vi "TestBed_NET.vi"() -> ()   [LabVIEW 2018]
uses:
  System.Net.Http
  <vilib>/httpClient/LabVIEWHTTPClient.lvlib
  <vilib>/httpClient/MultipartData.ctl
  <vilib>/addons/_JKI.lib/REST Client/classes/REST Client/REST Client.lvclass
panel:
  out "Numeric":i32
  out "Array 2":cluster{"Array":string[]}[](array[cluster])
  in  "ProxyAddress":string
  in  "String":string="https://reqres.in/api/users?page=2"
  out "Array":string[](array[string])
  out "Result":string
  out "StatusCode":i32(ring)=100 items=["Continue"=100, "SwitchingProtocols"=101, "OK"=200, "Created"=201, "Accepted"=202, "NonAuthoritativeInformation"=203, "NoContent"=204, "ResetContent"=205, "PartialContent"=206, "MultipleChoices, Ambiguous"=300, "MovedPermanently, Moved"=301, "Found, Redirect"=302, "SeeOther, RedirectMethod"=303, "NotModified"=304, "UseProxy"=305, "Unused"=306, "TemporaryRedirect, RedirectKeepVerb"=307, "BadRequest"=400, "Unauthorized"=401, "PaymentRequired"=402, "Forbidden"=403, "NotFound"=404, "MethodNotAllowed"=405, "NotAcceptable"=406, "ProxyAuthenticationRequired"=407, "RequestTimeout"=408, "Conflict"=409, "Gone"=410, "LengthRequired"=411, "PreconditionFailed"=412, "RequestEntityTooLarge"=413, "RequestUriTooLong"=414, "UnsupportedMediaType"=415, "RequestedRangeNotSatisfiable"=416, "ExpectationFailed"=417, "UpgradeRequired"=426, "InternalServerError"=500, "NotImplemented"=501, "BadGateway"=502, "ServiceUnavailable"=503, "GatewayTimeout"=504, "HttpVersionNotSupported"=505]
  # "http://httpbin.org/#/"
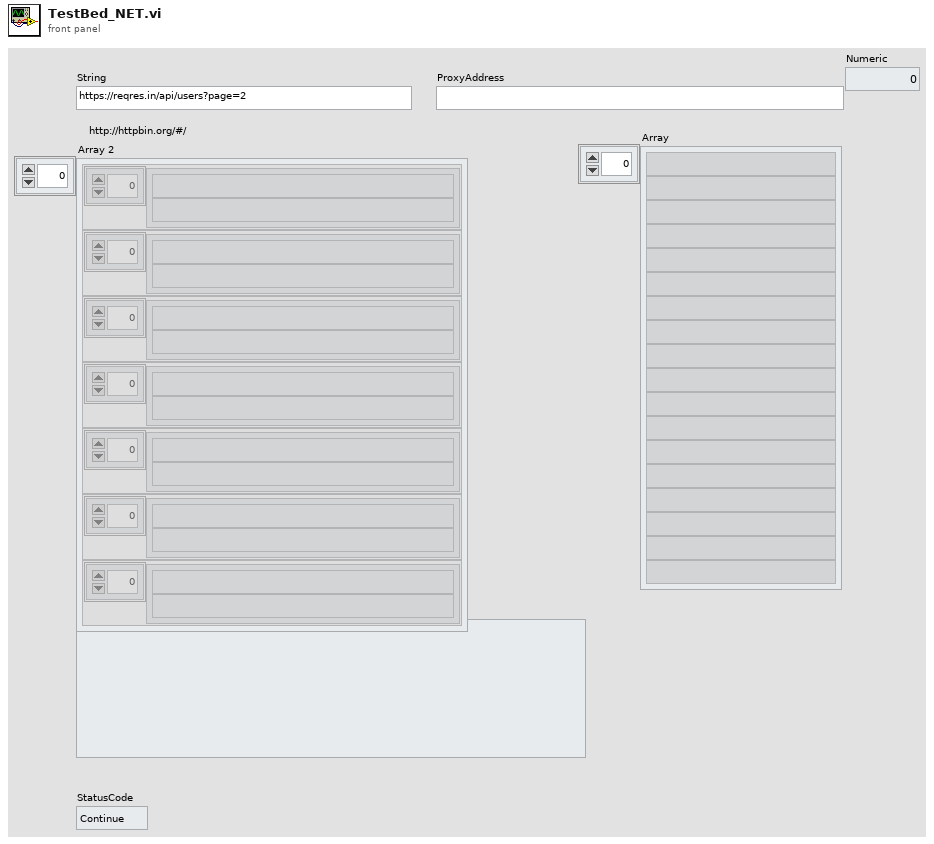
[diagram p1: front panel]
types:
  T1 = typedef "LabVIEWHTTPClient.lvlib/MultipartData.ctl" = cluster{"Name":string, "Value":string, "File":path, "Filename":string, "MIME type":string}
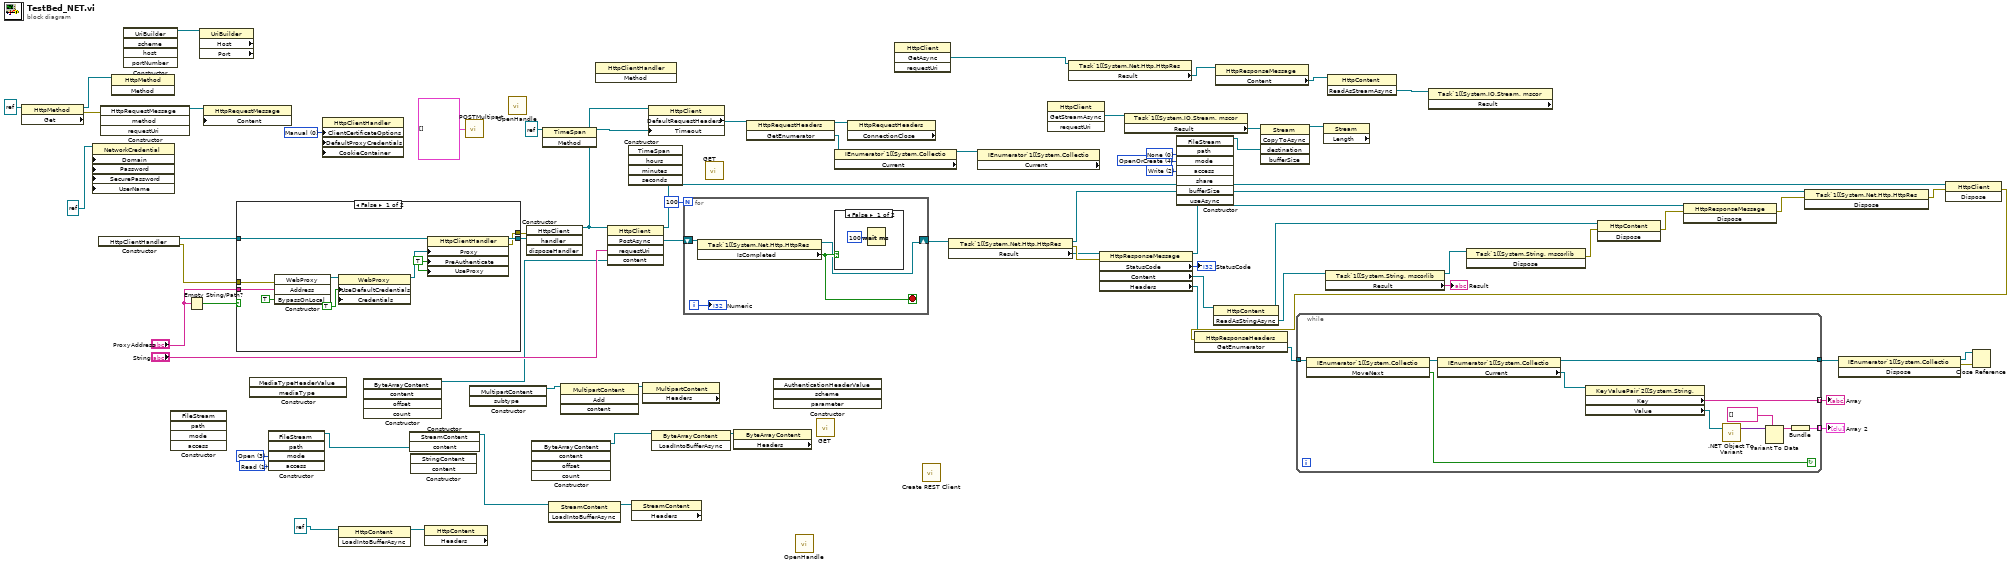
[diagram p0: block diagram]
diagram:
  w3 = 0 items=["None"=0, "Read"=1, "Write"=2, "ReadWrite"=3, "Delete"=4, "Inheritable"=16] ("share")
  w21 = 0 items=["Manual", "Automatic"] ("ClientCertificateOptions")
  w25 = 2 items=["Read"=1, "Write"=2, "ReadWrite"=3] ("access")
  w26 = 4 items=["CreateNew"=1, "Create"=2, "Open"=3, "OpenOrCreate"=4, "Truncate"=5, "Append"=6] ("mode")
  w31 = 1 items=["Read"=1, "Write"=2, "ReadWrite"=3] ("access")
  w32 = 3 items=["CreateNew"=1, "Create"=2, "Open"=3, "OpenOrCreate"=4, "Truncate"=5, "Append"=6] ("mode")
  n1 = property class="HttpMethod" props=["Get"](reference=refnum<k24> refnum) -> (reference out=w14:refnum<k24>, error out=w15:errorcluster)  [unwired: 1 in, 1 out]
  n2 = property class="NetworkCredential" props=["Domain", "Password", "SecurePassword", "UserName"](reference=refnum<k24> refnum ("cred")) -> ()  [unwired: 5 in, 2 out]
  n3 = constructor class="HttpClientHandler"() -> (reference out=w62:refnum<k24>, error out=w60:errorcluster)  [unwired: 3 in, 1 out]
  n4 = constructor class="HttpRequestMessage"(error in=w15) -> (reference out=w13:refnum<k24>)  [unwired: 4 in, 4 out]
  n5 = invoke class="HttpMethod" method=#-1(reference=w14) -> ()  [unwired: 2 in, 3 out]
  n6 = constructor class="UriBuilder"() -> (reference out=w6:refnum<k24>)  [unwired: 6 in, 5 out]
  n7 = constructor class="FileStream"() -> ()  [unwired: 6 in, 6 out]
  n8 = Empty String/Path?(string/path="ProxyAddress") -> (empty?=w58:bool)
  n9 = property class="UriBuilder" props=["Host", "Port"](reference=w6) -> ()  [unwired: 1 in, 4 out]
  n10 = property class="HttpRequestMessage" props=["Content"](reference=w13) -> ()  [unwired: 2 in, 2 out]
  n11 = case shown="False" w58 {
    tunnel: w62 -> [w81 w83]
    tunnel: [w80 w83] -> w61
    tunnel: w60 -> [w76 w82]
    tunnel: "ProxyAddress" -> [w75 _]
    tunnel: [w74 w82] -> w57
    frame False {
      w73 = TRUE ("PreAuthenticate")
      n12 = constructor class="WebProxy"(error in=w76, "Address"=w75, "BypassOnLocal"=TRUE) -> (reference out=w79:refnum<k24>)  [unwired: 2 in, 4 out]
      n13 = property class="WebProxy" props=["UseDefaultCredentials", "Credentials"](reference=w79, "UseDefaultCredentials"=TRUE) -> (reference out=w77:refnum<k24>)  [unwired: 2 in, 1 out]
      n14 = property class="HttpClientHandler"(reference=w81, "Proxy"=w77, "PreAuthenticate"=w73, "UseProxy"=w73) -> (reference out=w80:refnum<k24>, error out=w74:errorcluster)  [unwired: 1 in]
    }
    frame True {
    }
  }
  n15 = constructor class="MediaTypeHeaderValue"() -> ()  [unwired: 4 in, 4 out]
  n16 = constructor class="FileStream"("mode"=w32, "access"=w31) -> (reference out=w33:refnum<k24>)  [unwired: 4 in, 5 out]
  n17 = property class="HttpClientHandler" props=["ClientCertificateOptions", "DefaultProxyCredentials", "CookieContainer"]("ClientCertificateOptions"=w21) -> ()  [unwired: 4 in, 2 out]
  n18 = invoke class="HttpContent" method="LoadIntoBufferAsync"(reference=refnum<k24> refnum ("new reference")) -> (reference out=w8:refnum<k24>)  [unwired: 2 in, 2 out]
  n19 = constructor class="ByteArrayContent"() -> (reference out=w37:refnum<k24>)  [unwired: 6 in, 5 out]
  n20 = constructor class="StreamContent"("content"=w33) -> (reference out=w29:refnum<k24>)  [unwired: 3 in, 3 out]
  n21 = constructor class="StringContent"() -> ()  [unwired: 4 in, 4 out]
  n22 = property class="HttpContent" props=["Headers"](reference=w8) -> ()  [unwired: 1 in, 3 out]
  n23 = call <vilib>:"POSTMultipart.vi"("data"=T1[] []) -> ()  [unwired: 11 in, 4 out]
  n24 = constructor class="MultipartContent"() -> (reference out=w35:refnum<k24>)  [unwired: 4 in, 3 out]
  n25 = call <vilib>:"OpenHandle.vi"() -> ()  [unwired: 14 in, 2 out]
  n26 = constructor class="HttpClient"(error in=w57, "handler"=w61) -> (reference out=w19:refnum<k24>)  [unwired: 3 in, 4 out]
  n27 = constructor class="ByteArrayContent"() -> (reference out=w34:refnum<k24>)  [unwired: 6 in, 5 out]
  n28 = invoke class="TimeSpan" method=#-1(reference=refnum<k24> refnum ("Timeout")) -> (reference out=w11:refnum<k24>)  [unwired: 2 in, 2 out]
  n29 = invoke class="StreamContent" method="LoadIntoBufferAsync"(reference=w29) -> (reference out=w30:refnum<k24>)  [unwired: 2 in, 2 out]
  n30 = invoke class="MultipartContent" method="Add"(reference=w35) -> (reference out=w39:refnum<k24>)  [unwired: 3 in, 3 out]
  n31 = invoke class="HttpClientHandler" method=#-1() -> ()  [unwired: 3 in, 3 out]
  n32 = invoke class="HttpClient" method="PostAsync"(reference=w19, "requestUri"="String", "content"=w37) -> (reference out=w45:refnum<k24>, "PostAsync"=w43:refnum<k24>)  [unwired: 2 in, 3 out]
  n33 = constructor class="TimeSpan"() -> ()  [unwired: 6 in, 6 out]
  n34 = property class="StreamContent" props=["Headers"](reference=w30) -> ()  [unwired: 1 in, 3 out]
  n35 = property class="MultipartContent" props=["Headers"](reference=w39) -> ()  [unwired: 1 in, 3 out]
  n36 = property class="HttpClient"(reference=w19, "Timeout"=w11) -> ("DefaultRequestHeaders"=w18:refnum<k24>)  [unwired: 1 in, 2 out]
  n37 = invoke class="ByteArrayContent" method="LoadIntoBufferAsync"(reference=w34) -> (reference out=w38:refnum<k24>)  [unwired: 2 in, 2 out]
  n38 = for {
    N: 100 -> [_]
    shift-right: [w86] -> w41
    shift-left: w43 -> [w85]
    i -> [w84]
    stop <- w87 stop-if-true
    n39 = property class="Task`1[[System.Net.Http.HttpRes"(reference=w85) -> (reference out=w86:refnum<k24>, "IsCompleted"=w87:bool)  [unwired: 1 in, 1 out]
    n40 = case shown="False" w87 {
      frame False {
        n41 = Wait (ms)(milliseconds to wait=u32 100) -> ()  [unwired: 1 out]
      }
      frame True {
      }
    }
    "Numeric" <- w84
  }
  n42 = call <vilib>:"GET.vi"() -> ()  [unwired: 12 in, 4 out]
  n43 = property class="ByteArrayContent" props=["Headers"](reference=w38) -> ()  [unwired: 1 in, 3 out]
  n44 = invoke class="HttpRequestHeaders" method="GetEnumerator"(reference=w18) -> (reference out=w17:refnum<k24>, "GetEnumerator"=w10:refnum<k24>)  [unwired: 2 in, 1 out]
  n45 = constructor class="AuthenticationHeaderValue"() -> ()  [unwired: 5 in, 5 out]
  n46 = call <vilib>:"OpenHandle.vi"() -> ()  [unwired: 14 in, 2 out]
  n47 = call <vilib>:"GET.vi"() -> ()  [unwired: 12 in, 4 out]
  n48 = property class="IEnumerator`1[[System.Collectio" props=["Current"](reference=w10) -> (reference out=w9:refnum<k24>)  [unwired: 1 in, 2 out]
  n49 = property class="HttpRequestHeaders" props=["ConnectionClose"](reference=w17) -> ()  [unwired: 1 in, 3 out]
  n50 = invoke class="HttpClient" method="GetAsync"() -> ("GetAsync"=w24:refnum<k24>)  [unwired: 4 in, 3 out]
  n51 = call <vilib>:"Create REST Client.vi"() -> ()  [unwired: 10 in, 2 out]
  n52 = property class="Task`1[[System.Net.Http.HttpRes"(reference=w41) -> (reference out=w48:refnum<k24>, error out=w70:errorcluster, "Result"=w69:refnum<k24>)  [unwired: 1 in]
  n53 = property class="IEnumerator`1[[System.Collectio" props=["Current"](reference=w9) -> ()  [unwired: 1 in, 3 out]
  n54 = invoke class="HttpClient" method="GetStreamAsync"() -> ("GetStreamAsync"=w28:refnum<k24>)  [unwired: 4 in, 3 out]
  n55 = property class="Task`1[[System.Net.Http.HttpRes"(reference=w24) -> ("Result"=w23:refnum<k24>)  [unwired: 1 in, 2 out]
  n56 = property class="HttpResponseMessage"(reference=w69, error in=w70) -> (reference out=w50:refnum<k24>, "StatusCode"=→"StatusCode":i32, "Content"=w67:refnum<k24>, "Headers"=w5:refnum<k24>)  [unwired: 1 out]
  n57 = property class="Task`1[[System.IO.Stream, mscor"(reference=w28) -> ("Result"=w27:refnum<k24>)  [unwired: 1 in, 2 out]
  n58 = constructor class="FileStream"("mode"=w26, "access"=w25, "share"=w3) -> (reference out=w1:refnum<k24>)  [unwired: 6 in, 8 out]
  n59 = invoke class="HttpContent" method="ReadAsStringAsync"(reference=w67) -> (reference out=w51:refnum<k24>, "ReadAsStringAsync"=w66:refnum<k24>)  [unwired: 2 in, 1 out]
  n60 = property class="HttpResponseMessage"(reference=w23) -> ("Content"=w22:refnum<k24>)  [unwired: 1 in, 2 out]
  n61 = invoke class="Stream" method="CopyToAsync"(reference=w27, "destination"=w1) -> (reference out=w2:refnum<k24>)  [unwired: 3 in, 4 out]
  n62 = property class="Stream" props=["Length"](reference=w2) -> ()  [unwired: 1 in, 3 out]
  n63 = property class="Task`1[[System.String, mscorlib"(reference=w66) -> (reference out=w53:refnum<k24>, "Result"=→"Result":string)  [unwired: 1 in, 1 out]
  n64 = invoke class="HttpContent" method="ReadAsStreamAsync"(reference=w22) -> ("ReadAsStreamAsync"=w4:refnum<k24>)  [unwired: 2 in, 2 out]
  n65 = property class="Task`1[[System.IO.Stream, mscor" props=["Result"](reference=w4) -> ()  [unwired: 1 in, 3 out]
  n66 = invoke class="Task`1[[System.String, mscorlib" method="Dispose"(reference=w53) -> (error out=w52:errorcluster)  [unwired: 2 in, 2 out]
  n67 = invoke class="HttpContent" method="Dispose"(reference=w51, error in=w52) -> (error out=w49:errorcluster)  [unwired: 1 in, 2 out]
  n68 = invoke class="HttpResponseMessage" method="Dispose"(reference=w50, error in=w49) -> (error out=w47:errorcluster)  [unwired: 1 in, 2 out]
  n69 = invoke class="Task`1[[System.Net.Http.HttpRes" method="Dispose"(reference=w48, error in=w47) -> (error out=w46:errorcluster)  [unwired: 1 in, 2 out]
  n70 = invoke class="HttpClient" method="Dispose"(reference=w45, error in=w46) -> (error out=w40:errorcluster)  [unwired: 1 in, 2 out]
  n71 = invoke class="HttpResponseHeaders" method="GetEnumerator"(reference=w5, error in=w40) -> ("GetEnumerator"=w64:refnum<k24>)  [unwired: 1 in, 2 out]
  n72 = while {
    tunnel: w64 -> [w99]
    tunnel: [w97] -> w63 mode=indexing
    tunnel: [w89] -> w44 mode=indexing
    tunnel: [w90] -> w56
    stop <- w91 continue-if-true
    n73 = invoke class="IEnumerator`1[[System.Collectio" method="MoveNext"(reference=w99) -> (reference out=w96:refnum<k24>, "MoveNext"=w91:bool)  [unwired: 2 in, 1 out]
    n74 = property class="IEnumerator`1[[System.Collectio"(reference=w96) -> (reference out=w90:refnum<k24>, "Current"=w98:refnum<k24>)  [unwired: 1 in, 1 out]
    n75 = property class="KeyValuePair`2[[System.String, "(reference=w98) -> ("Key"=w97:string, "Value"=w95:refnum<k24>)  [unwired: 1 in, 2 out]
    n76 = call <vilib>:".NET Object To Variant.vi"(".NET object"=w95) -> ("variant"=w94:variant)  [unwired: 1 in, 1 out]
    n77 = Variant To Data(type=string[] [], Variant=w94) -> (data=w92:string[])  [unwired: 1 in, 1 out]
    n78 = Bundle(w92) -> (w89:cluster{string[]})  [unwired: 1 in]
  }
  "Array" <- w63
  "Array 2" <- w44
  n79 = invoke class="IEnumerator`1[[System.Collectio" method="Dispose"(reference=w56) -> (reference out=w54:refnum<k24>, error out=w55:errorcluster)  [unwired: 2 in, 1 out]
  n80 = Close Reference(reference=w54, error in (no error)=w55) -> ()  [unwired: 1 out]
